vi "Init Test Result Data.vi"(8 "error in (no error)":errorcluster, 10 "Test Result.lvclass":refnum<class "Test Result.lvclass">, 11 "Measure in":refnum<class "Measure.lvclass">) -> (0 "error out":errorcluster, 3 "Measure out":refnum<class "Measure.lvclass">)   [LabVIEW 2021, in "Sequence Engine.lvlib" / "Measure.lvclass"]
uses:
  Measure.lvclass
  Test Result/Test Result.lvclass
  Measure.lvclass/Measure.ctl
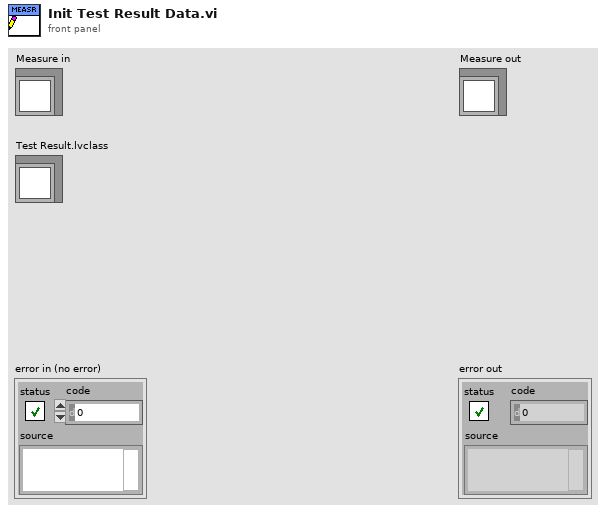
[diagram p1: front panel]
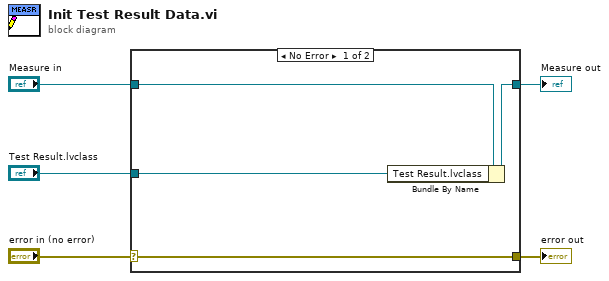
[diagram p0: block diagram]
diagram:
  n1 = case shown="No Error" "error in (no error)" {
    selector: "error in (no error)" -> [w9 w10]
    tunnel: [w9 w10] -> w4
    tunnel: [w7 w11] -> w2
    tunnel: "Measure in" -> [w8 w11]
    tunnel: "Test Result.lvclass" -> [w6 _]
    frame No Error {
      n2 = Bundle By Name(cluster=w8, "Test Result.lvclass"=w6) -> (w7:refnum<class "Measure.lvclass">)
    }
    frame Error {
    }
  }
  "error out" <- w4
  "Measure out" <- w2
